vi "Nctp Ramp Done.vi"(4 "Close Received":bool, 5 "MCL State In":T1, 6 "error in":errorcluster, 7 "Stop Requests":T2, 9 "MCL Cmd In":refnum<queue>) -> (0 "error out":errorcluster, 2 "NTCP MM Finish State":T3, 3 "MCL Cmd Out":refnum<queue>)   [LabVIEW 2013]
uses:
  NTCP Client/MM 2 NTCP Message.ctl
  NTCP library/NTCP Commands.ctl
  Apps/Yes No Button.ctl
  NTCP Mixed Mode States.ctl
  Stop Requests.ctl
  MCL Done Or Abort.ctl
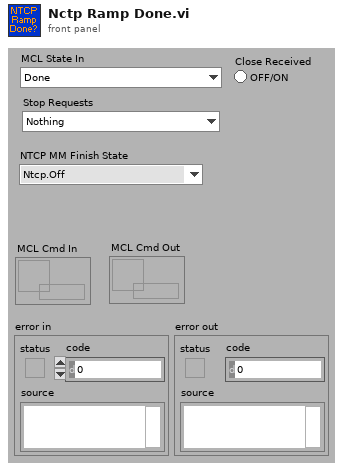
[diagram p1: front panel]
types:
  T1 = typedef "MCL Done Or Abort.ctl" = enum16{"Done", "Abort", "Still Running"}
  T2 = typedef "Stop Requests.ctl" = enum16{"Nothing", "Stop Requested", "Abort Requested"}
  T3 = typedef "NTCP Mixed Mode States.ctl" = enum16{"Ntcp.Off", "Ntcp.WaitForProposal", "Ntcp.WaitForAccept", "Ntcp.WaitForExecute", "Ntcp.WaitForStart", "Ntcp.WaitForMclRamp", "Ntcp.WaitForMclDone", "Ntcp.Shutdown"}
  T4 = typedef "MM 2 NTCP Message.ctl" = cluster{"NTCP commands":T5, "Transaction ID":string, "Control Point":string, "Accepted":T6}
  T5 = typedef "NTCP Commands.ctl" = enum16{"propose", "execute", "cancel", "set-parameter", "get-parameter", "open-session", "close-session", "get-control-point", "Unknown", "stop"}
  T6 = typedef "Yes No Button.ctl" = bool
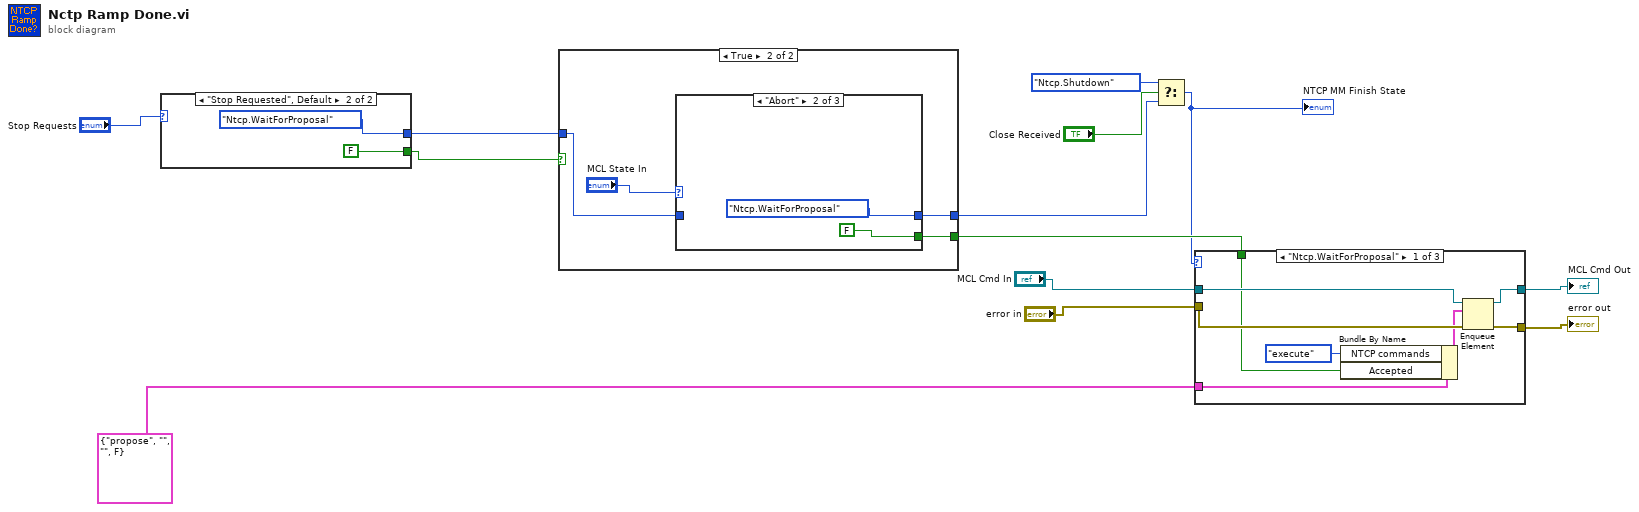
[diagram p0: block diagram]
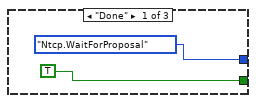
[diagram p3: hidden frame]
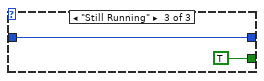
[diagram p4: hidden frame]
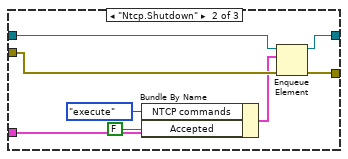
[diagram p5: hidden frame]
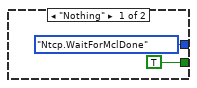
[diagram p7: hidden frame]
diagram:
  n1 = case shown="\"Stop Requested\", Default" "Stop Requests" {
    tunnel: [NTCP_Mixed_Mode_States."Ntcp.WaitForMclDone" ("NTCP MM States") NTCP_Mixed_Mode_States."Ntcp.WaitForProposal" ("NTCP MM States")] -> w3
    tunnel: [TRUE FALSE] -> w1
    frame "Nothing" {
    }
    frame "Stop Requested", Default {
    }
  }
  n2 = case shown="True" w1 {
    selector: w1 -> [w19 _]
    tunnel: [w19 w20] -> w13
    tunnel: [w18 w23] -> w4
    tunnel: w3 -> [w18 w22]
    frame False {
    }
    frame True {
      n3 = case shown="\"Abort\"" "MCL State In" {
        tunnel: [NTCP_Mixed_Mode_States."Ntcp.WaitForProposal" ("NTCP MM States") NTCP_Mixed_Mode_States."Ntcp.WaitForProposal" ("NTCP MM States") w29] -> w23
        tunnel: w22 -> [_ _ w29]
        tunnel: [TRUE FALSE TRUE] -> w20
        frame "Done" {
        }
        frame "Abort" {
        }
        frame "Still Running" {
        }
      }
    }
  }
  n4 = Select(t=NTCP_Mixed_Mode_States."Ntcp.Shutdown", s="Close Received", f=w4) -> (s? t:f=w7:T3)
  "NTCP MM Finish State" <- w7
  n5 = case shown="\"Ntcp.WaitForProposal\"" w7 {
    tunnel: T4 {"NTCP commands"=enum."propose", "Transaction ID"="", "Control Point"="", "Accepted"=FALSE} ("NTCP Message") -> [w37 w45 _]
    tunnel: "MCL Cmd In" -> [w35 w42 w47]
    tunnel: [w34 w41 w47] -> w10
    tunnel: "error in" -> [w33 w40 w46]
    tunnel: [w32 w39 w46] -> w12
    tunnel: w13 -> [w30 _ _]
    frame "Ntcp.WaitForProposal" {
      n6 = Bundle By Name(cluster=w37, "NTCP commands"=NTCP_Commands."execute", "Accepted"=w30) -> (w31:T4)
      n7 = Enqueue Element(queue=w35, element=w31, error in (no error)=w33) -> (queue out=w34:refnum<queue>, error out=w32:errorcluster)  [unwired: 1 in, 1 out]
    }
    frame "Ntcp.Shutdown" {
      n8 = Bundle By Name(cluster=w45, "NTCP commands"=NTCP_Commands."execute", "Accepted"=T6 FALSE) -> (w38:T4)
      n9 = Enqueue Element(queue=w42, element=w38, error in (no error)=w40) -> (queue out=w41:refnum<queue>, error out=w39:errorcluster)  [unwired: 1 in, 1 out]
    }
    frame "Ntcp.WaitForMclDone", Default {
    }
  }
  "error out" <- w12
  "MCL Cmd Out" <- w10
